vi "readErrorOrWarnings.vi"(8 "error in (no error)":errorcluster, 9 "typeOfError":T1, 10 "id":T2=1, 11 "CoolerControler in":refnum<class "CoolerControler.lvclass">) -> (0 "error out":errorcluster, 2 "errorsArray":u16[](array[numeric]), 3 "CoolerControler out":refnum<class "CoolerControler.lvclass">)   [LabVIEW 2016, in "CoolerControler.lvclass"]
uses:
  CoolerControler.lvclass
  typedefs/CoolerId.ctl
  typedefs/typeOfError.ctl
  SerialCommand/CoolerSerialCommand.lvclass
  typedefs/CoolerQuery.ctl
  typedefs/errorType.ctl
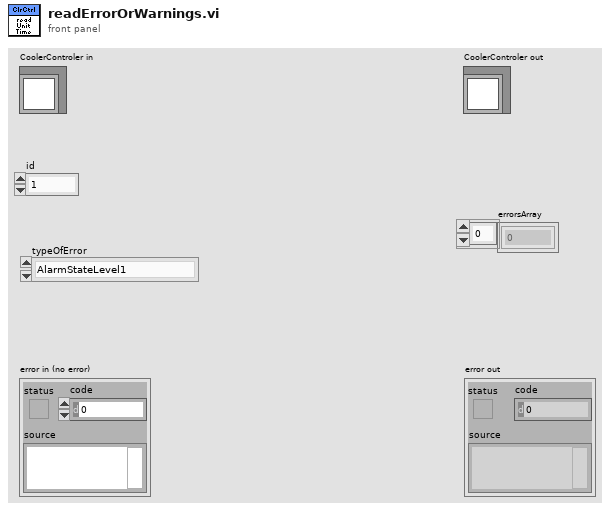
[diagram p1: front panel]
types:
  T1 = typedef "typeOfError.ctl" = enum16{"AlarmStateLevel1", "AlarmStateLevel21", "AlarmStateLevel22", "WarningStateLevel1"}
  T2 = typedef "CoolerId.ctl" = u16
  T3 = typedef "CoolerQuery.ctl" = enum16{"ReadSerialWatchdog", "ReadControlSensor", "ReadSetTemperature", "ReadSupplyTemperature", "ReadExternalRTD", "ReadExternalThermistor", "ReadReturnTemperature", "ReadAmbientTemperature", "ReadProcessFlow", "ReadTECBank1Current", "ReadTECBank2Current", "ReadTEDriveLevel", "ReadAlarmStateLevel1", "ReadAlarmStateLevel21", "ReadAlarmStateLevel22", "ReadWarningStateLevel1", "ReadHighSupplyTempWarning", "ReadLowSupplyTempWarning", "ReadHighAmbientTempWarning", "ReadLowAmbientTempWarning", "ReadLowProcessFlowWarning", "ReadHighSupplyTempAlarm", "ReadLowSupplyTempAlarm", "ReadHighAmbientTempAlarm", "ReadLowAmbientTempAlarm", "ReadLowProcessFlowAlarm", "ReadPWMandRelayStatus", "ReadPIDStatus", "ReadUnitUpTime", "ReadFan1Speed", "ReadFan2Speed", "ReadFan3Speed", "ReadFan4Speed"}
  T4 = typedef "response.ctl" = cluster{"deviceId":string, "commandNumber":string, "errorActive":bool, "commandName":string, "responseData":string, "checkSum":string}
  T5 = typedef "errorType.ctl" = cluster{"type":enum16{"AlarmStateLevel1", "AlarmStateLevel21", "AlarmStateLevel22", "WarningStateLevel1"}, "errorValue":u16}
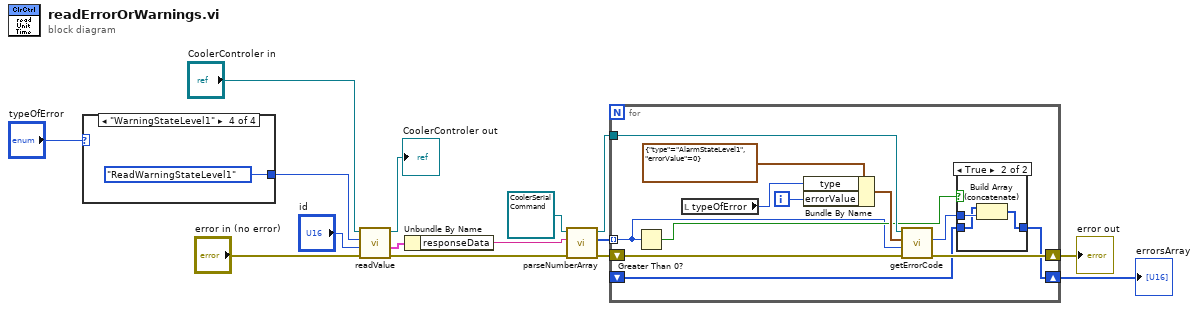
[diagram p0: block diagram]
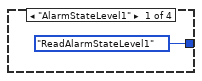
[diagram p3: hidden frame]
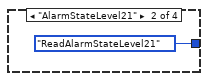
[diagram p4: hidden frame]
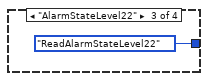
[diagram p5: hidden frame]
diagram:
  n1 = case shown="\"WarningStateLevel1\"" "typeOfError" {
    tunnel: [CoolerQuery."ReadAlarmStateLevel1" ("CoolerQuery") CoolerQuery."ReadAlarmStateLevel21" ("CoolerQuery") CoolerQuery."ReadAlarmStateLevel22" ("CoolerQuery") CoolerQuery."ReadWarningStateLevel1" ("CoolerQuery")] -> w12
    frame "AlarmStateLevel1" {
    }
    frame "AlarmStateLevel21" {
    }
    frame "AlarmStateLevel22" {
    }
    frame "WarningStateLevel1" {
    }
  }
  n2 = call "readValue.vi"("error in (no error)"="error in (no error)", "id"="id", "CoolerQuery"=w12, "CoolerControler in"="CoolerControler in") -> ("error out"=w7:errorcluster, "response out"=w10:T4, "CoolerControler out"=→"CoolerControler out":refnum<class "CoolerControler.lvclass">)  [unwired: 4 in, 1 out]
  n3 = Unbundle By Name(w10) -> ("responseData"=w6:string)
  n4 = call "parseNumberArray.vi"("error in (no error)"=w7, "commandData"=w6, "CoolerSerialCommand in"=refnum<class "CoolerSerialCommand.lvclass"> refnum) -> ("error out"=w3:errorcluster, "NumberArray"=w4:u16[], "CoolerSerialCommand out"=w5:refnum<class "CoolerSerialCommand.lvclass">)  [unwired: 6 in]
  n5 = for {
    tunnel: w5 -> [w31]
    tunnel: w4 -> [w21] mode=indexing
    shift-right: [w27] -> w2
    shift-left: w3 -> [w28]
    shift-right: [w23] -> w1
    shift-left: _ -> [w20]
    i -> [w26]
    n6 = Greater Than 0?(x=w21) -> (x > 0?=w22:bool)
    n7 = local read "typeOfError"() -> (w30:T1)
    n8 = Bundle By Name(cluster=T5 {"type"=enum."AlarmStateLevel1", "errorValue"=0} ("errorType"), "type"=w30, "errorValue"=w26) -> (w25:T5)
    n9 = call "getErrorCode.vi"("error in (no error)"=w28, "code"=w21, "errorType"=w25, "CoolerSerialCommand in"=w31) -> ("error out"=w27:errorcluster, "errorCode"=w24:u16)  [unwired: 5 in, 1 out]
    n10 = case shown="True" w22 {
      tunnel: w24 -> [_ w35]
      tunnel: [w32 w34] -> w23
      tunnel: w20 -> [w32 w33]
      frame False {
      }
      frame True {
        n11 = Build Array (concatenate)(w33, w35) -> (w34:u16[])
      }
    }
  }
  "error out" <- w2
  "errorsArray" <- w1
